vi "Gaussian_Quantiles.vi"(8 "error in (no error)":errorcluster caption="entrée d'erreur (pas d'erreur)", 11 "make_gaussian_quantiles":T2={"mean"=[-1.0], "cov "=1.0, "n_samples"=100, "n_features"=2, "n_classes"=3, "shuffle"=TRUE, "random_state"=-1, "Returns"="X"} {"random_state" min=-1; "n_classes" min=1; "n_features" min=1; "n_samples" min=1}) -> (0 "error out":errorcluster, 3 "Data":T1)   [LabVIEW 2020]
doc: "Generate isotropic Gaussian and label samples by quantile\n\nThis classification dataset is constructed by taking a multi-dimensional standard normal distribution and defining classes separated by nested concentric multi-dimensional spheres such that roughly equal numbers of samples are in each class (quantiles of the distribution).\n\n\n\nParameters :\n\n- mean : array of shape [n_features], optional (default=None=-1)\nThe mean of the multi-dimensional normal distribution. If None then use the origin (0, 0, …).\n\n- cov : float, optional (default=1.)\nThe covariance matrix will be this value times the unit matrix. This dataset only produces symmetric normal distributions.\n\n- n_samples : int, optional (default=100)\nThe total number of points equally divided among classes.\n\n- n_features : int, optional (default=2)\nThe number of features for each sample.\n\n- n_classes : int, optional (default=3)\nThe number of classes\n\n- shuffle : boolean, optional (default=True)\nShuffle the samples.\n\n- random_state : int, RandomState instance, default=None=-1\nDetermines random number generation for dataset creation. Pass an int for reproducible output across multiple function calls. See Glossary.\n\nReturns : \n\n- X : array of shape [n_samples, n_features]\nThe generated samples.\n\n- y : array of shape [n_samples]\nThe integer labels for quantile membership of each sample."
uses:
  Gaussian_Quantiles.lvclass
panel:
  out "Gaussian_Quantiles.lvclass":refnum<class "Gaussian_Quantiles.lvclass">
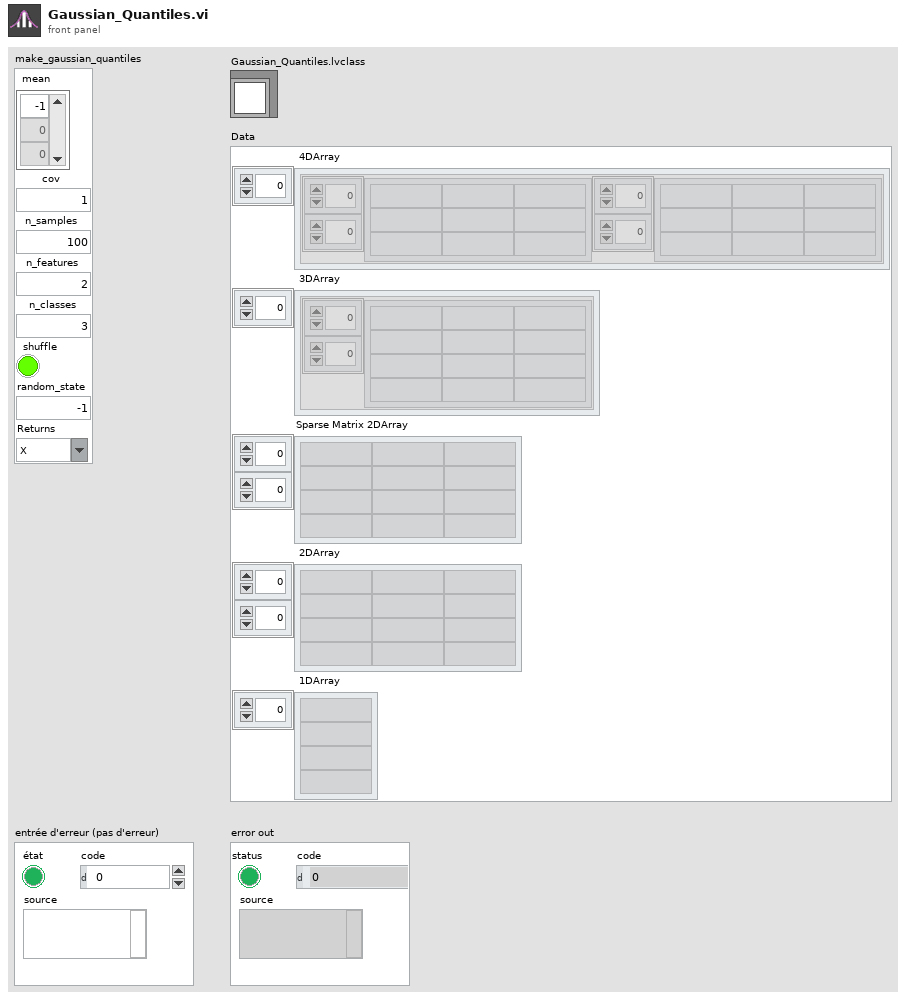
[diagram p1: front panel]
types:
  T1 = cluster{" 4DArray":cluster{"1":string[][], "2":string[][]}[], " 3DArray":cluster{"Tableau":string[][]}[], "Sparse Matrix 2DArray":string[][], " 2DArray":string[][], " 1DArray":string[]}
  T2 = cluster{"mean":dbl[], "cov ":dbl, "n_samples":u32, "n_features":u32, "n_classes":u32, "shuffle":bool, "random_state":i32, "Returns":string}
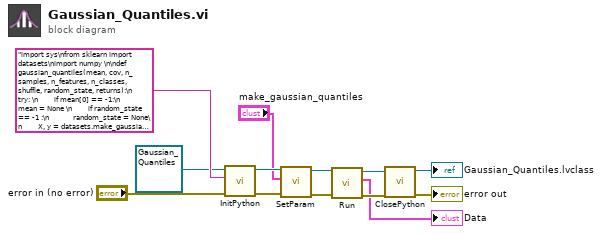
[diagram p0: block diagram]
diagram:
  n1 = call-dynamic "InitPython.vi"("error in (no error)"="error in (no error)", "Python Instruction"="import sys\nfrom sklearn import datasets\nimport numpy \n\ndef gaussian_quantiles(mean, cov, n_samples, n_features, n_classes, shuffle, random_state, returns):\n    try: \n        if mean[0] == -1:\n            mean = None \n        if random_state == -1 :\n            random_state = None\n        X, y = datasets.make_gaussian_quantiles(mean, cov, n_samples, n_features, n_classes, shuffle, random_state)\n        if returns == 'X':\n            dataX = X.tolist()\n            return str(dataX)\n        else :\n            datay = y.tolist()\n            return str(datay)\n    except:\n        erreur = sys.exc_info()\n        typerr = u\"%s\" % (erreur[0])\n        typerr = typerr[typerr.find(\"'\")+1:typerr.rfind(\"'\")]\n        msgerr = u\"%s\" % (erreur[1])\n        message = str('/!\\\\ {0} : {1}'. format(typerr,msgerr))\n        return message", "Scikit-learn en entrée"=refnum<class "Gaussian_Quantiles.lvclass"> refnum ("Gaussian_Quantiles.lvclass")) -> ("error out"=w9:errorcluster, "Scikit-learn en sortie"=w10:refnum<class "Gaussian_Quantiles.lvclass">)  [unwired: 7 in]
  n2 = call-dynamic "SetParam.vi"("error in (no error)"=w9, "make_gaussian_quantiles"="make_gaussian_quantiles", "Gaussian_Quantiles.lvclass"=w10) -> ("error out"=w6:errorcluster, "Gaussian_Quantiles.lvclass"=w7:refnum<class "Gaussian_Quantiles.lvclass">)  [unwired: 7 in]
  n3 = call-dynamic "Run.vi"("error in (no error)"=w6, "Gaussian_Quantiles.lvclass"=w7) -> ("error out"=w4:errorcluster, "Data"=→"Data":T1, "Gaussian_Quantiles.lvclass"=w5:refnum<class "Gaussian_Quantiles.lvclass">)  [unwired: 7 in]
  n4 = call-dynamic "ClosePython.vi"("error in (no error)"=w4, "Scikit-learn en entrée"=w5) -> ("error out"=→"error out":errorcluster, "Scikit-learn en sortie"=→"Gaussian_Quantiles.lvclass":refnum<class "Gaussian_Quantiles.lvclass">)  [unwired: 8 in]
